vi "Hatch Panel Intake.vi"   [LabVIEW 2018]
uses:
  <vilib>/Rock Robotics/WPI/Solenoid/WPI_SolenoidChannel.ctl
  <vilib>/Rock Robotics/WPI/Solenoid/WPI_SolenoidValue.ctl
  Hatch Panel Intake Global.vi
  <vilib>/Rock Robotics/WPI/Solenoid/WPI_SolenoidOpenSingle.vi
  Controllers/Manipulator Controlller/Manipulator Controller Global.vi
  <vilib>/Rock Robotics/WPI/Solenoid/WPI_SolenoidSetEnum.vi
  Cargo Intake/Cargo Intake Global.vi
  Times/Times Global.vi
types:
  T1 = typedef "WPI_SolenoidChannel.ctl" = enum8{"Solenoid 0", "Solenoid 1", "Solenoid 2", "Solenoid 3", "Solenoid 4", "Solenoid 5", "Solenoid 6", "Solenoid 7", "Invalid"}
  T2 = enum16{"Full Manual Control", "Manual Control", "Autonomous Control", "Fully Autonomous Control"}
  T3 = typedef "WPI_SolenoidValue.ctl" = enum16{"Off", "On", "Forward", "Reverse"}
  T4 = typedef "WPI_SolenoidDevRef.ctl" = cluster{"DevStatus":errorcluster, "Pneumatics Control Module":u8, "Forward Solenoid Channel":T1, "Reverse Solenoid Channel":T1}
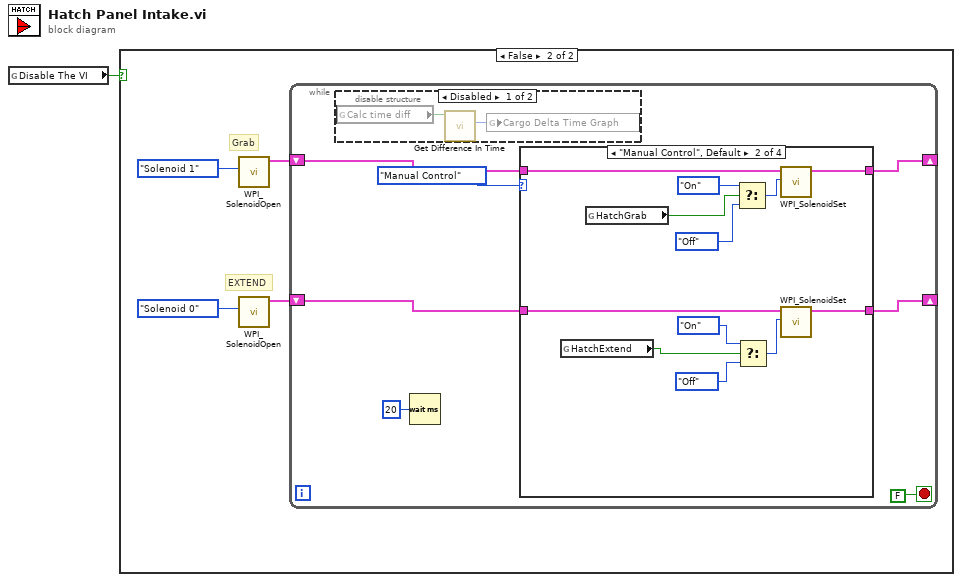
[diagram p0: block diagram]
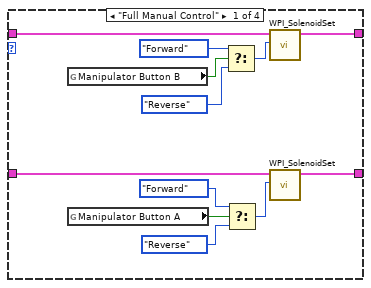
[diagram p4: hidden frame]
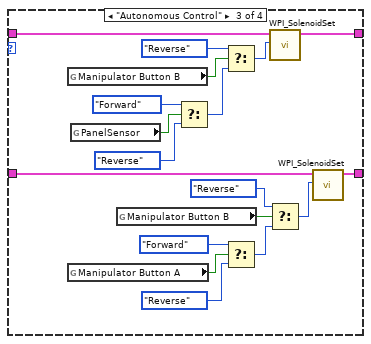
[diagram p5: hidden frame]
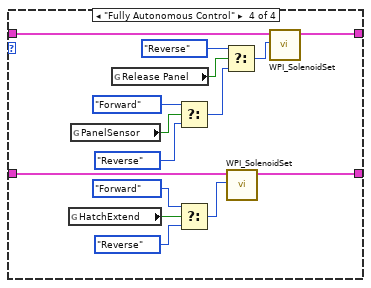
[diagram p6: hidden frame]
diagram:
  n1 = global read "Hatch Panel Intake Global.vi" "Disable The VI"() -> (w1:bool)
  n2 = case shown="False" w1 {
    frame True {
    }
    frame False {
      # "EXTEND"
      # "Grab"
      n3 = call-poly <vilib>:"WPI_SolenoidOpen.vi"("Solenoid Channel"=WPI_SolenoidChannel."Solenoid 1" ("Forward Solenoid Channel")) -> ("SolenoidDevRef"=w2:T4)  [unwired: 9 in, 1 out]
      n4 = call-poly <vilib>:"WPI_SolenoidOpen.vi"("Solenoid Channel"=WPI_SolenoidChannel."Solenoid 0" ("Forward Solenoid Channel")) -> ("SolenoidDevRef"=w5:T4)  [unwired: 9 in, 1 out]
      n5 = while {
        shift-right: [w8] -> _
        shift-left: w2 -> [w9]
        shift-right: [w7] -> _
        shift-left: w5 -> [w10]
        stop <- FALSE stop-if-true
        n6 = disable-structure shown="Disabled" {
          frame Disabled {
            n7 = global read "Cargo Intake Global.vi" "Calc time diff"() -> (w14:bool)
            n8 = call "Get Difference In Time.vi"("Calculate Time Difference"=w14) -> ("Delta Time over Time"=w13:u32)  [unwired: 9 in, 1 out]
            n9 = global write "Times Global.vi" "Cargo Delta Time Graph"(w13) -> ()
          }
          frame Enabled {
          }
        }
        n10 = Wait (ms)(milliseconds to wait=u32 20) -> ()  [unwired: 1 out]
        n11 = case shown="\"Manual Control\", Default" T2."Manual Control" ("Mode") {
          tunnel: w10 -> [w18 w33 w54 w69]
          tunnel: w9 -> [w17 w32 w56 w70]
          tunnel: [w15 w30 w55 w71] -> w8
          tunnel: [w16 w31 w53 w68] -> w7
          frame "Full Manual Control" {
            n12 = global read "Manipulator Controller Global.vi" "Manipulator Button B"() -> (w20:bool)
            n13 = global read "Manipulator Controller Global.vi" "Manipulator Button A"() -> (w23:bool)
            n14 = Select(t=WPI_SolenoidValue."Forward" ("Value"), s=w20, f=WPI_SolenoidValue."Reverse" ("Value")) -> (s? t:f=w19:T3)
            n15 = Select(t=WPI_SolenoidValue."Forward" ("Value"), s=w23, f=WPI_SolenoidValue."Reverse" ("Value")) -> (s? t:f=w24:T3)
            n16 = call-poly <vilib>:"WPI_SolenoidSet.vi"("Value"=w19, "SolenoidDevRef"=w17) -> ("SolenoidDevRef"=w15:T4)  [unwired: 8 in, 1 out]
            n17 = call-poly <vilib>:"WPI_SolenoidSet.vi"("Value"=w24, "SolenoidDevRef"=w18) -> ("SolenoidDevRef"=w16:T4)  [unwired: 8 in, 1 out]
          }
          frame "Manual Control", Default {
            n18 = global read "Hatch Panel Intake Global.vi" "HatchExtend"() -> (w27:bool)
            n19 = global read "Hatch Panel Intake Global.vi" "HatchGrab"() -> (w28:bool)
            n20 = Select(t=WPI_SolenoidValue."On" ("Value"), s=w28, f=WPI_SolenoidValue."Off" ("Value")) -> (s? t:f=w34:T3)
            n21 = Select(t=WPI_SolenoidValue."On" ("Value"), s=w27, f=WPI_SolenoidValue."Off" ("Value")) -> (s? t:f=w37:T3)
            n22 = call-poly <vilib>:"WPI_SolenoidSet.vi"("Value"=w34, "SolenoidDevRef"=w32) -> ("SolenoidDevRef"=w30:T4)  [unwired: 8 in, 1 out]
            n23 = call-poly <vilib>:"WPI_SolenoidSet.vi"("Value"=w37, "SolenoidDevRef"=w33) -> ("SolenoidDevRef"=w31:T4)  [unwired: 8 in, 1 out]
          }
          frame "Autonomous Control" {
            n24 = global read "Manipulator Controller Global.vi" "Manipulator Button B"() -> (w52:bool)
            n25 = global read "Manipulator Controller Global.vi" "Manipulator Button A"() -> (w40:bool)
            n26 = global read "Hatch Panel Intake Global.vi" "PanelSensor"() -> (w51:bool)
            n27 = global read "Manipulator Controller Global.vi" "Manipulator Button B"() -> (w44:bool)
            n28 = Select(t=WPI_SolenoidValue."Forward" ("Value"), s=w51, f=WPI_SolenoidValue."Reverse" ("Value")) -> (s? t:f=w50:T3)
            n29 = Select(t=WPI_SolenoidValue."Reverse", s=w52, f=w50) -> (s? t:f=w46:T3)
            n30 = Select(t=WPI_SolenoidValue."Forward" ("Value"), s=w40, f=WPI_SolenoidValue."Reverse" ("Value")) -> (s? t:f=w41:T3)
            n31 = call-poly <vilib>:"WPI_SolenoidSet.vi"("Value"=w46, "SolenoidDevRef"=w56) -> ("SolenoidDevRef"=w55:T4)  [unwired: 8 in, 1 out]
            n32 = Select(t=WPI_SolenoidValue."Reverse" ("Value"), s=w44, f=w41) -> (s? t:f=w39:T3)
            n33 = call-poly <vilib>:"WPI_SolenoidSet.vi"("Value"=w39, "SolenoidDevRef"=w54) -> ("SolenoidDevRef"=w53:T4)  [unwired: 8 in, 1 out]
          }
          frame "Fully Autonomous Control" {
            n34 = global read "Hatch Panel Intake Global.vi" "HatchExtend"() -> (w58:bool)
            n35 = global read "Hatch Panel Intake Global.vi" "PanelSensor"() -> (w65:bool)
            n36 = global read "Hatch Panel Intake Global.vi" "Release Panel"() -> (w62:bool)
            n37 = Select(t=WPI_SolenoidValue."Forward" ("Value"), s=w65, f=WPI_SolenoidValue."Reverse" ("Value")) -> (s? t:f=w64:T3)
            n38 = Select(t=WPI_SolenoidValue."Forward" ("Value"), s=w58, f=WPI_SolenoidValue."Reverse" ("Value")) -> (s? t:f=w59:T3)
            n39 = Select(t=WPI_SolenoidValue."Reverse", s=w62, f=w64) -> (s? t:f=w63:T3)
            n40 = call-poly <vilib>:"WPI_SolenoidSet.vi"("Value"=w59, "SolenoidDevRef"=w69) -> ("SolenoidDevRef"=w68:T4)  [unwired: 8 in, 1 out]
            n41 = call-poly <vilib>:"WPI_SolenoidSet.vi"("Value"=w63, "SolenoidDevRef"=w70) -> ("SolenoidDevRef"=w71:T4)  [unwired: 8 in, 1 out]
          }
        }
      }
    }
  }
